vi "Write CSV File_1D (UTF-16).vi"(7 "delimiter (,) *ASCII":string=",", 8 "error in (no error)":errorcluster, 9 "append to file? (new file)":bool, 10 "1D array *UTF-16":string[](array[string]), 11 "file path in":path) -> (0 "error out":errorcluster, 3 "file path out":path)   [LabVIEW 2013, in "SET_Robust CSV (UTF-16).lvlib"]
doc: "Write a single CSV record to CSV file. The CSV file is formatted in accordance with RFC-4180 (see http://tools.ietf.org/html/rfc4180). \n\nA custom delimiter character can be specified. Default is a comma.\n\nSetting \"append to file?\" to true will append a single record to the end of an existing file. Setting \"append to file?\" to false will overwrite an existing file. In both cases, if the file is not found, a new file will be created.\n\nRev 0.0 2014-02-20 Ryan Porter\nFirst Draft"
uses:
  SET_Robust CSV (UTF-16).lvlib
panel:
  # "Write CSV File_1D.vi\n\nWrite a single CSV record to CSV file. The CSV file is formatted in accordance with RFC-4180 (see http://tools.ietf.org/html/rfc4180). \n\nA custom delimiter character can be specified. Default is a comma.\n\nSetting \"append to file?\" to true will append a single record to the end of an existing file. Setting \"append to file?\" to false will overwrite an existing file. In both cases, if the file is not found, a new file will be created."
  # "License: BSD (2-Clause) - http://opensource.org/licenses/BSD-2-Clause \n\nCopyright (c) 2014, Ryan Porter\nAll rights reserved."
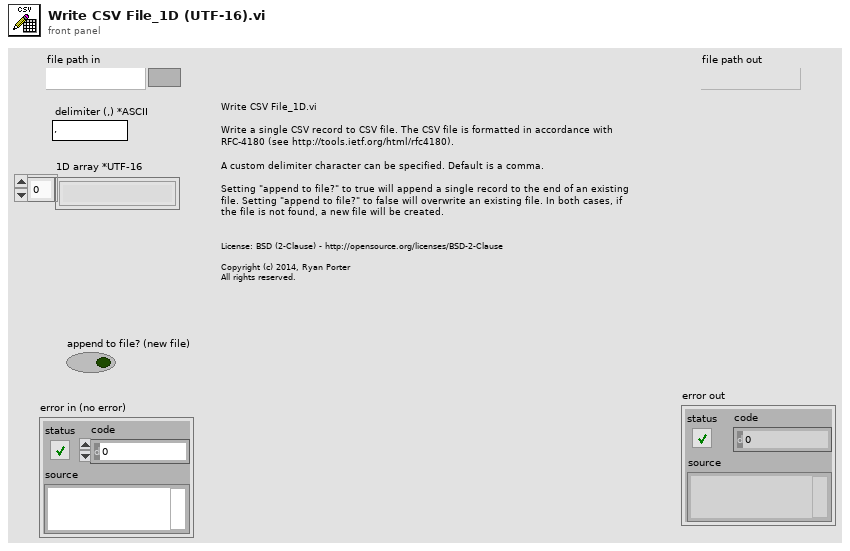
[diagram p1: front panel]
types:
  T1 = enum16{"open", "replace", "create", "open or create", "replace or create", "replace or create with confirmation"}
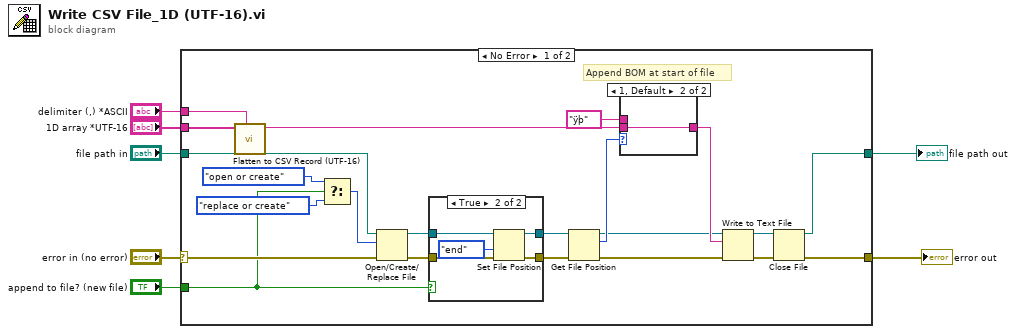
[diagram p0: block diagram]
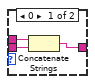
[diagram p2: hidden frame]
diagram:
  n1 = case shown="No Error" "error in (no error)" {
    selector: "error in (no error)" -> [w29 w42]
    tunnel: "1D array *UTF-16" -> [w17 _]
    tunnel: "delimiter (,) *ASCII" -> [w16 _]
    tunnel: [w20 w42] -> w4
    tunnel: "file path in" -> [w28 w41]
    tunnel: "append to file? (new file)" -> [w22 _]
    tunnel: [w18 w41] -> w1
    frame No Error {
      # "Append BOM at start of file"
      n2 = call "Flatten to CSV Record (UTF-16).vi"("delimiter (,) *ASCII"=w16, "row of strings *UTF-16"=w17) -> ("CSV record *UTF-16"=w12:string)  [unwired: 8 in, 1 out]
      n3 = Select(t=T1."open or create" ("operation (0:open)"), s=w22, f=T1."replace or create" ("operation (0:open)")) -> (s? t:f=w25:T1)
      n4 = Open/Create/Replace File(file path (use dialog)=w28, error in=w29, operation (0:open)=w25) -> (refnum out=w24:refnum<file>, error out=w23:errorcluster)  [unwired: 3 in, 1 out]
      n5 = case shown="True" w22 {
        tunnel: w24 -> [w35 w40]
        tunnel: w23 -> [w34 w39]
        tunnel: [w34 w37] -> w14
        tunnel: [w35 w36] -> w15
        frame False {
        }
        frame True {
          n6 = Set File Position(refnum=w40, from (0:start)=enum16{"start", "end", "current"}."end", error in=w39) -> (refnum out=w36:refnum<file>, error out=w37:errorcluster)  [unwired: 1 in]
        }
      }
      n7 = Get File Position(4:w14, 7:w15) -> (0:w10:errorcluster, 2:w13:i64, 3:w9:refnum<file>)
      n8 = case shown="1, Default" w13 {
        tunnel: w12 -> [w32 w33]
        tunnel: [w31 w33] -> w11
        tunnel: "ÿþ" -> [w30 _]
        frame 0 {
          n9 = Concatenate Strings(w30, w32) -> (w31:string)
        }
        frame 1, Default {
        }
      }
      n10 = Write to Text File(file (use dialog)=w9, text=w11, error in=w10) -> (refnum out=w19:refnum<file>, error out=w21:errorcluster)  [unwired: 1 in, 1 out]
      n11 = Close File(refnum=w19, error in=w21) -> (path=w18:path, error out=w20:errorcluster)
    }
    frame Error {
    }
  }
  "error out" <- w4
  "file path out" <- w1
